vi "Retrieve Ringdown Data.vi"(8 "error in":errorcluster, 11 "cCRDS in":refnum<class "cCRDS.lvclass">) -> (0 "error out":errorcluster, 3 "cCRDS out":refnum<class "cCRDS.lvclass">)   [LabVIEW 2015, in "cCRDS.lvclass"]
uses:
  cCRDS.lvclass
  cCRDS.lvclass/cCRDS.ctl
  Reusable/CRDS/Main/CRDS.lvclass/CRDS.ctl
  <vilib>/DAQmx/read.llb/DAQmx Read (Analog 2D I16 NChan NSamp).vi
  Data Access/Read Laser Cfg.vi
  Reusable/CRDS/Main/Write Laser Data.vi
  new/Data Access/Read AI.vi
  Reusable/CRDS/Main/Read Cells.vi
  <vilib>/DAQmx/miscellaneous.llb/DAQmx Fill In Error Info.vi
  Reusable/CRDS/Cell/CRDS Cell.lvclass
  <resource>/objmgr/daqmx.rc
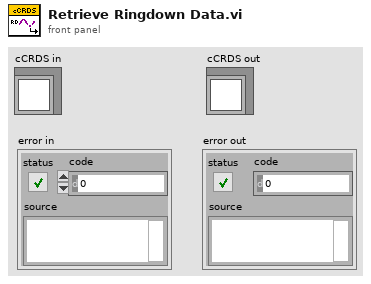
[diagram p1: front panel]
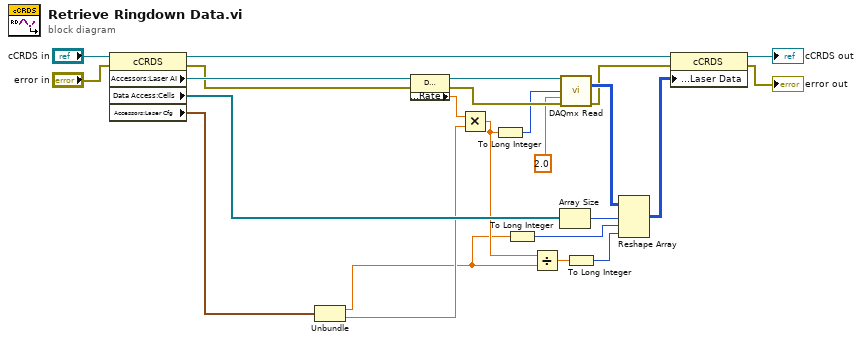
[diagram p0: block diagram]
diagram:
  n1 = property class="cCRDS"(reference="cCRDS in", error in="error in") -> (reference out=w15:refnum<class "cCRDS.lvclass">, error out=w12:errorcluster, "Accessors:Laser AI"=w17:refnum<k21>, "Data Access:Cells"=w13:refnum<class "CRDS Cell.lvclass">[], "Accessors:Laser Cfg"=w3:cluster{"Rate (Hz)":sgl, "DC (%)":sgl})
  n2 = Unbundle(w3) -> ("Rate (Hz)"=w1:sgl, "DC (%)"=w2:sgl)
  n3 = property class="DAQmx Timing"(reference=w17, error in=w12) -> (reference out=w10:refnum<k21>, error out=w21:errorcluster, "SampClk.Rate"=w9:dbl)
  n4 = Multiply(x=w9, y=w2) -> (x*y=w8:dbl)
  n5 = To Long Integer(number=w8) -> (32bit integer=w20:i32)
  n6 = To Long Integer(number=w1) -> (32bit integer=w4:i32)
  n7 = Divide(x=w8, y=w1) -> (x/y=w19:dbl)
  n8 = Array Size(array=w13) -> (size(s)=w23:i32)
  n9 = call-poly <vilib>:"DAQmx Read.vi"("task/channels in"=w10, "number of samples per channel"=w20, "timeout"=2.0, "error in"=w21) -> ("data"=w22:i16[][], "error out"=w7:errorcluster)  [unwired: 10 out]
  n10 = To Long Integer(number=w19) -> (32bit integer=w5:i32)
  n11 = Reshape Array(w22, w23, w4, w5) -> (w6:i16[][][])
  n12 = property class="cCRDS"(reference=w15, error in=w7, "Data Access:Laser Data"=w6) -> (reference out=→"cCRDS out":refnum<class "cCRDS.lvclass">, error out=→"error out":errorcluster)
